vi "Folders整体图.vi"() -> ()   [LabVIEW 2014]
panel:
  in  "Mail":bool
  in  "Lock":bool
  in  "Important":bool
  in  "Image":bool
  in  "Home":bool
  in  "Help":bool
  in  "Games":bool
  in  "Font":bool
  in  "Folder":bool
  in  "Favorite":bool
  in  "Download":bool
  in  "Audio":bool
  in  "Video":bool
  in  "Text":bool
  in  "Print":bool
  in  "Photo":bool
  in  "Package":bool
  in  "Open":bool
  in  "New":bool
  in  "Network":bool
  in  "Navigation":bool
  in  "Media":bool
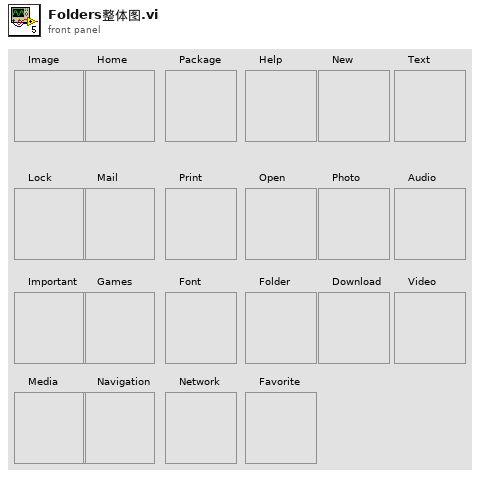
[diagram p1: front panel]
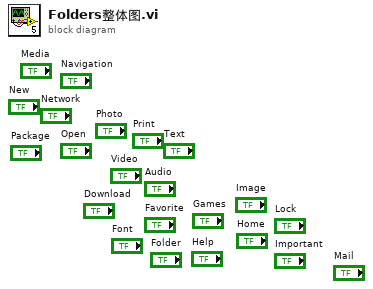
[diagram p0: block diagram]
diagram:
